vi "SQLite Gen Std.PKWhere Statement.vi"(8 "error in":errorcluster, 11 "Cluster in":refnum<vi>) -> (0 "error out":errorcluster, 3 "delimited string":string)   [LabVIEW 2021, in "EDT SQLite+.lvlib"]
uses:
  EDT SQLite+.lvlib
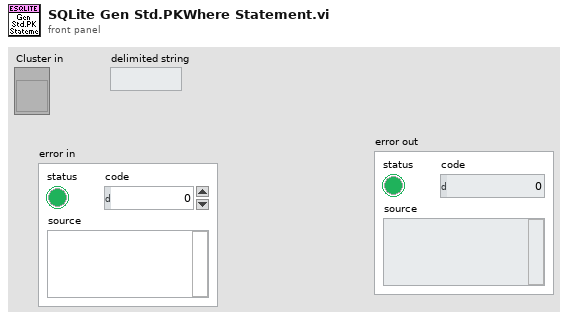
[diagram p1: front panel]
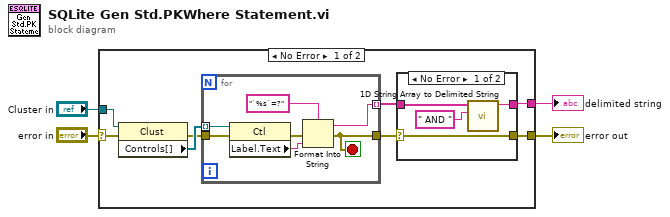
[diagram p0: block diagram]
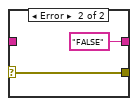
[diagram p2: hidden frame]
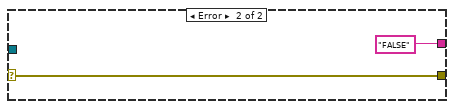
[diagram p3: hidden frame]
diagram:
  n1 = case shown="No Error" "error in" {
    selector: "error in" -> [w8 w27]
    tunnel: [w11 "FALSE" ("delimited string")] -> w4
    tunnel: "Cluster in" -> [w9 _]
    tunnel: [w5 w27] -> w1
    frame No Error {
      n2 = property class="Clust"(reference=w9, error in=w8) -> (error out=w7:errorcluster, "Controls[]"=w12:refnum<vi>[])  [unwired: 1 out]
      n3 = for {
        tunnel: w12 -> [w25] mode=indexing
        tunnel: [w22] -> w10 mode=indexing
        tunnel: w7 -> [w21]
        tunnel: [w19] -> w6
        stop <- w19 stop-if-true
        n4 = property class="Ctl"(reference=w25, error in=w21) -> (error out=w20:errorcluster, "Label.Text"=w24:string)  [unwired: 1 out]
        n5 = Format Into String(format string="`%s`=?", error in=w20, w24) -> (resulting string=w22:string, error out=w19:errorcluster)  [unwired: 1 in]
      }
      n6 = case shown="No Error" w6 {
        selector: w6 -> [w13 w17]
        tunnel: [w16 "FALSE" ("delimited string")] -> w11
        tunnel: w10 -> [w14 _]
        tunnel: [w13 w17] -> w5
        frame No Error {
          n7 = call <vilib>:"1D String Array to Delimited String.vi"("delimiter"=" AND ", "string array"=w14) -> ("delimited string"=w16:string)  [unwired: 9 in]
        }
        frame Error {
        }
      }
    }
    frame Error {
    }
  }
  "delimited string" <- w4
  "error out" <- w1
